vi "Tab Controls Disabled.vi"(6 "Page":i32, 8 "Disabled":u8, 11 "Tab Control Pages":refnum<vi>[](array[refnum])) -> ()   [LabVIEW 2016]
doc: "This VI sets the Disabled property of all controls on the selected page of the specified tab control."
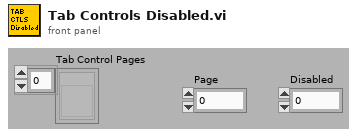
[diagram p1: front panel]
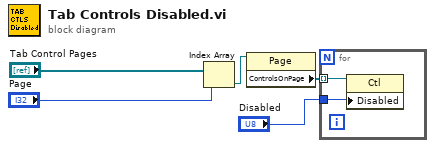
[diagram p0: block diagram]
diagram:
  n1 = Index Array(array="Tab Control Pages", index="Page") -> (element=w4:refnum<vi>)
  n2 = property class="Page"(reference=w4) -> ("ControlsOnPage"=w5:refnum<vi>[])  [unwired: 1 in, 2 out]
  n3 = for {
    tunnel: w5 -> [w7] mode=indexing
    tunnel: "Disabled" -> [w6]
    n4 = property class="Ctl"(reference=w7, "Disabled"=w6) -> ()  [unwired: 1 in, 2 out]
  }
